vi "mircuz.vi"() -> (3 "x":dbl)   [LabVIEW 2019]
uses:
  <vilib>/Rock Robotics/Network Tables/NT Read Number.vi
  Robot Global Data.vi
panel:
  in  "x 2":dbl=-0.01
  in  "x":dbl=0.18
  in  "p":dbl=0.02
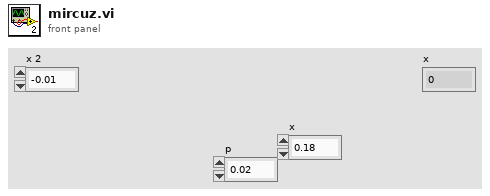
[diagram p1: front panel]
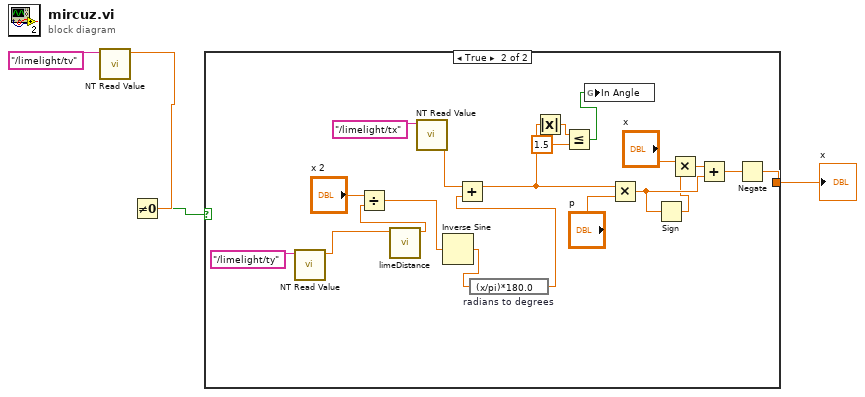
[diagram p0: block diagram]
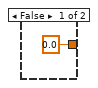
[diagram p2: hidden frame]
diagram:
  n1 = call-poly <vilib>:"NT Read Value.vi"("Name"="/limelight/tv") -> ("Numeric"=w2:dbl)  [unwired: 9 in, 1 out]
  n2 = Not Equal To 0?(x=w2) -> (x != 0?=w1:bool)
  n3 = case shown="True" w1 {
    tunnel: [0.0 w7] -> w4
    frame False {
    }
    frame True {
      n4 = call-poly <vilib>:"NT Read Value.vi"("Name"="/limelight/ty") -> ("Numeric"=w17:dbl)  [unwired: 9 in, 1 out]
      n5 = call "limeDistance.vi"("a2"=w17) -> ("d"=w16:dbl)  [unwired: 10 in]
      n6 = Divide(x="x 2", y=w16) -> (x/y=w15:dbl)
      n7 = call-poly <vilib>:"NT Read Value.vi"("Name"="/limelight/tx") -> ("Numeric"=w19:dbl)  [unwired: 9 in, 1 out]
      n8 = Inverse Sine(1:w15) -> (0:w14:dbl)
      n9 = expression code="(x/pi)*180.0" "radians to degrees"(w14) -> (w13:dbl)
      n10 = Add(x=w19, y=w13) -> (x+y=w12:dbl)
      n11 = Absolute Value(x=w12) -> (abs(x)=w11:dbl)
      n12 = Less Or Equal?(x=w11, y=1.5) -> (x <= y?=w9:bool)
      n13 = global write "Robot Global Data.vi" "In Angle"(w9) -> ()
      n14 = Multiply(x=w12, y="p") -> (x*y=w23:dbl)
      n15 = Sign(1:w23) -> (0:w8:dbl)
      n16 = Multiply(x="x", y=w8) -> (x*y=w21:dbl)
      n17 = Add(x=w21, y=w23) -> (x+y=w20:dbl)
      n18 = Negate(x=w20) -> (-x=w7:dbl)
    }
  }
  "x" <- w4
